vi "SystemLink_Write_Boolean.vi"(9 "Boolean":bool, 11 "SL_XControl":T1(xcontrol)) -> ()   [LabVIEW 2019]
uses:
  SL_XControl.xctl
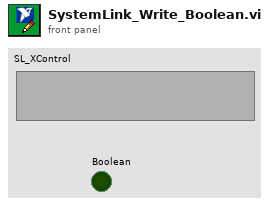
[diagram p1: front panel]
types:
  T1 = cluster{"Tag":string, "Type":string, "Data":string}
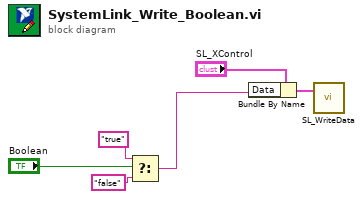
[diagram p0: block diagram]
diagram:
  n1 = Select(t="true", s="Boolean", f="false") -> (s? t:f=w6:string)
  n2 = Bundle By Name(cluster="SL_XControl", "Data"=w6) -> (w4:T1)
  n3 = call "SL_WriteData.vi"("Tag"=w4) -> ()  [unwired: 11 in]
